vi "Destroy.vi"(0 "reference in":refnum<class "Master Controller.lvclass">, 5 "error in (no error)":errorcluster) -> (14 "reference out":refnum<class "Master Controller.lvclass">, 19 "error out":errorcluster)   [LabVIEW 2015, in "Master Controller.lvclass"]
doc: "Destructor."
uses:
  Master Controller.lvclass
  <vilib>/addons/_AddQ/G#Object/G#Object.lvclass
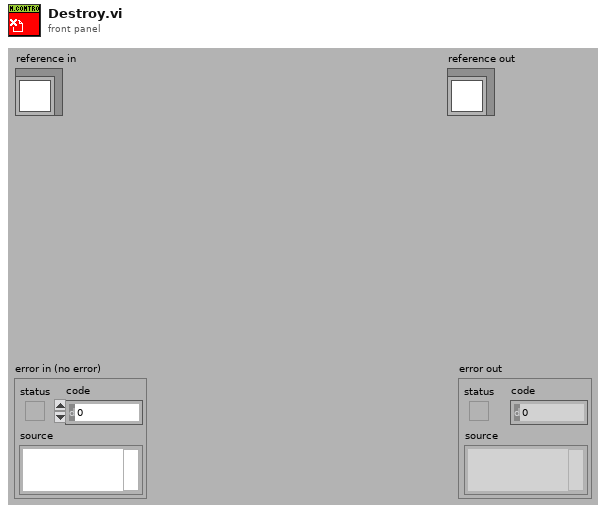
[diagram p1: front panel]
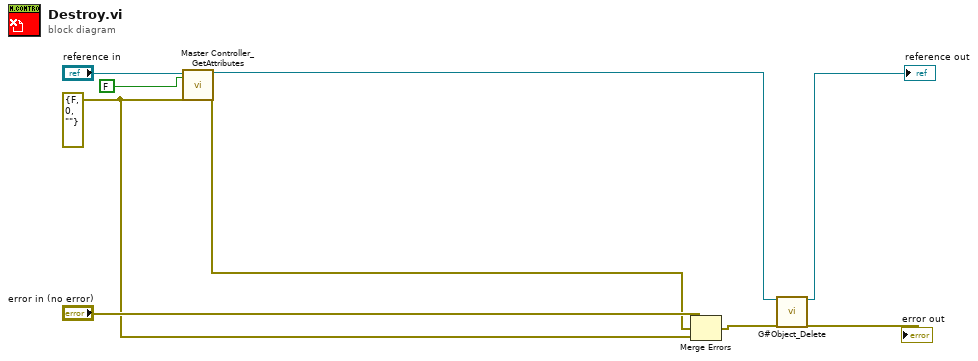
[diagram p0: block diagram]
diagram:
  w6 = errorcluster {"status"=FALSE, "code"=0, "source"=""} ("error in (no error)")
  n1 = call "Master Controller_GetAttributes.vi"("reference in"="reference in", "return data? (T)"=FALSE ("simple info"), "error in (no error)"=w6) -> ("reference out"=w3:refnum<class "Master Controller.lvclass">, "error out"=w8:errorcluster)  [unwired: 13 in, 2 out]
  n2 = Merge Errors("error in (no error)", w8, w6) -> (w5:errorcluster)
  n3 = call <vilib>:"G#Object_Delete.vi"("reference in"=w3, "error in (no error)"=w5) -> ("reference out"=→"reference out":refnum<class "Master Controller.lvclass">, "error out"=→"error out":errorcluster)  [unwired: 16 in]
